vi "scan frame corner.vi"(0 "Speed (m/s)":dbl=1e-09 format="%#_6p", 1 "Corner (T = top left, F = bottom left)":bool) -> ()   [LabVIEW 2021]
uses:
  <userlib>/Nanonis Prog Interface V5/Nanonis Prog Interface.lvlib
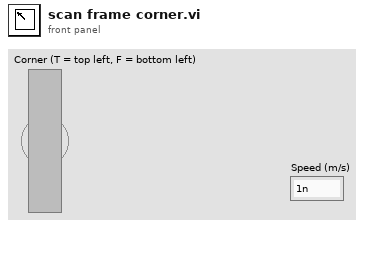
[diagram p1: front panel]
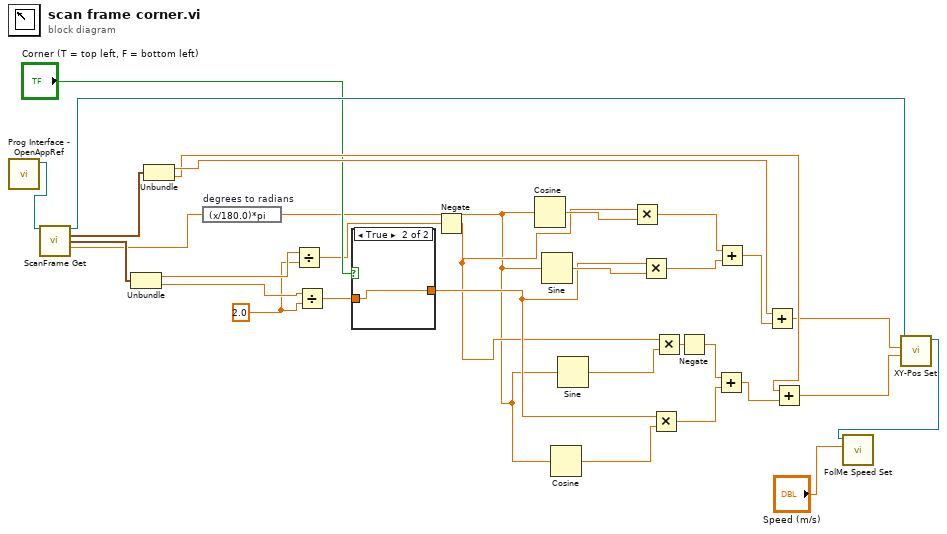
[diagram p0: block diagram]
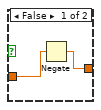
[diagram p2: hidden frame]
diagram:
  w18 = sgl 2.0 ("y")
  n1 = call <userlib>:"Prog Interface - OpenAppRef.vi"() -> ("Application reference"=w26:refnum<vi>)  [unwired: 6 in, 1 out]
  n2 = call <userlib>:"ScanFrame Get.vi"("Application ref in"=w26) -> ("Application ref out"=w25:refnum<vi>, "Center coordinates (m)"=w31:cluster{"Xc":sgl, "Yc":sgl}, "Size (m)"=w30:cluster{"Width":sgl, "Height":sgl}, "Angle (deg)"=w27:sgl)  [unwired: 10 in, 1 out]
  n3 = Unbundle(w30) -> ("Width"=w29:sgl, "Height"=w28:sgl)
  n4 = Unbundle(w31) -> ("Xc"=w22:sgl, "Yc"=w21:sgl)
  n5 = expression code="(x/180.0)*pi" "degrees to radians"(w27) -> (w5:sgl)
  n6 = Divide(x=w29, y=w18) -> (x/y=w8:sgl)
  n7 = Divide(x=w28, y=w18) -> (x/y=w11:sgl)
  n8 = case shown="True" "Corner (T = top left, F = bottom left)" {
    tunnel: w11 -> [w33 w34]
    tunnel: [w32 w34] -> w10
    frame False {
      n9 = Negate(x=w33) -> (-x=w32:sgl)
    }
    frame True {
    }
  }
  n10 = Negate(x=w8) -> (-x=w6:sgl)
  n11 = Cosine(x=w5) -> (cos(x)=w17:sgl)
  n12 = Sine(x=w5) -> (sin(x)=w16:sgl)
  n13 = Cosine(x=w5) -> (cos(x)=w13:sgl)
  n14 = Sine(x=w5) -> (sin(x)=w14:sgl)
  n15 = Multiply(x=w6, y=w17) -> (x*y=w15:sgl)
  n16 = Multiply(x=w10, y=w16) -> (x*y=w4:sgl)
  n17 = Multiply(x=w10, y=w13) -> (x*y=w12:sgl)
  n18 = Multiply(x=w6, y=w14) -> (x*y=w7:sgl)
  n19 = Negate(x=w7) -> (-x=w3:sgl)
  n20 = Add(x=w3, y=w12) -> (x+y=w24:sgl)
  n21 = Add(x=w15, y=w4) -> (x+y=w23:sgl)
  n22 = Add(x=w22, y=w23) -> (x+y=w20:sgl)
  n23 = Add(x=w21, y=w24) -> (x+y=w19:sgl)
  n24 = call <userlib>:"XY-Pos Set.vi"("Y (m)"=w19, "X (m)"=w20, "Application ref in"=w25) -> ("Application ref out"=w1:refnum<vi>)  [unwired: 5 in, 1 out]
  n25 = call <userlib>:"FolMe Speed Set.vi"("Speed (m/s)"="Speed (m/s)", "Application ref in"=w1) -> ()  [unwired: 6 in, 2 out]
